vi "Set Expected Heartbeat Entry.vi"(8 "error in":errorcluster, 9 "Entry":T1 {"Last Beat" format="%<%x %.3X>T"; "Timeout" format="%d ms"; "Period" format="%d ms"}, 10 "Node-ID":u8, 11 "Network Management UI in":refnum<class "Network Management UI.lvclass">) -> (0 "error out":errorcluster, 3 "Network Management UI out":refnum<class "Network Management UI.lvclass">)   [LabVIEW 2020, in "Network Management UI.lvlib" / "Network Management UI.lvclass"]
uses:
  Network Management UI.lvclass
  Network Management UI.lvclass/Network Management UI.ctl
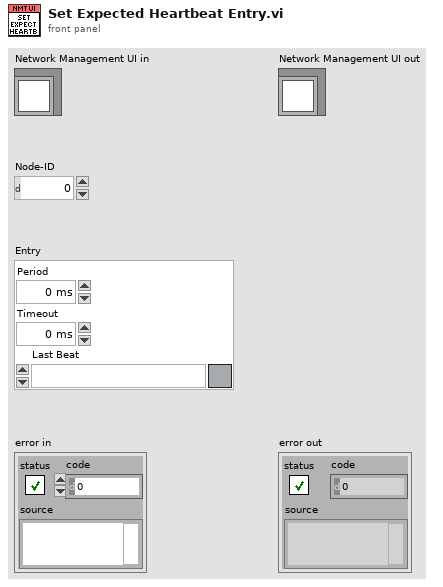
[diagram p1: front panel]
types:
  T1 = cluster{"Period":u16, "Timeout":u16, "Last Beat":timestamp}
  T2 = map{u8, cluster{"Period":u16, "Timeout":u16, "Last Beat":timestamp}}
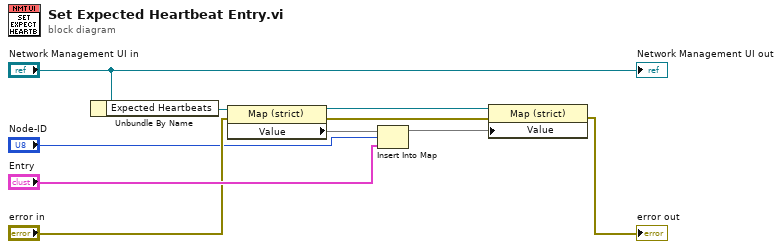
[diagram p0: block diagram]
diagram:
  n1 = Unbundle By Name("Network Management UI in") -> ("Expected Heartbeats"=w9:refnum<vi>)
  n2 = property class="Map (strict)"(reference=w9, error in="error in") -> (reference out=w5:refnum<vi>, error out=w3:errorcluster, "Value"=w8:T2)
  n3 = Insert Into Map(map in=w8, key="Node-ID", value="Entry") -> (map out=w4:T2)  [unwired: 2 out]
  n4 = property class="Map (strict)"(reference=w5, error in=w3, "Value"=w4) -> (error out=→"error out":errorcluster)  [unwired: 1 out]
  "Network Management UI out" <- "Network Management UI in"
